vi "Update Status.vi"(9 "Spec Page Interface":T1, 11 "TwoTasksMetaDataObj in":refnum<class "DCAFConfigurablePluginDecideFeatures.lvclass">) -> ()   [LabVIEW 2013, in "DCAFConfigurablePluginDecideFeatures.lvclass"]
uses:
  DCAFConfigurablePluginDecideFeatures.lvclass
  <resource>/dialog/NewProjectWizard/Spec Page Interface.ctl
  <resource>/dialog/NewProjectWizard/MetaDataObj/MetaDataObj.lvclass/MetaDataObj.ctl
  <resource>/dialog/NewProjectWizard/MetaDataObj/Accessors/Read Project Name.vi
  <resource>/dialog/NewProjectWizard/MetaDataObj/Accessors/Read Project Root.vi
  <resource>/dialog/NewProjectWizard/MetaDataObj/Accessors/Read File Prefix.vi
panel:
  in  "Please choose a different name.":string="Please choose a different name."
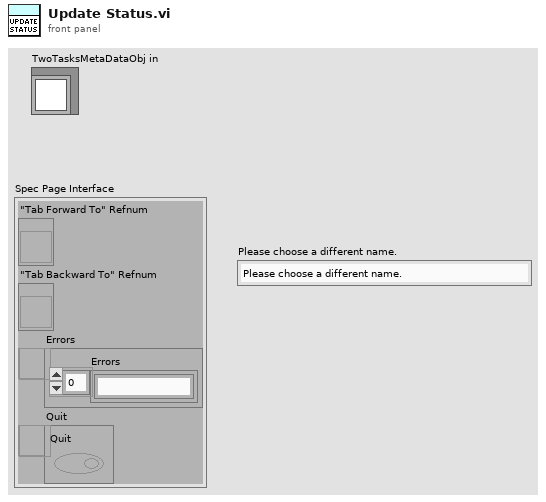
[diagram p1: front panel]
types:
  T1 = typedef "Spec Page Interface.ctl" = cluster{"\"Tab Forward To\" Refnum":refnum<vi>, "\"Tab Backward To\" Refnum":refnum<vi>, "Errors":refnum<user-event>, "Quit":refnum<user-event>}
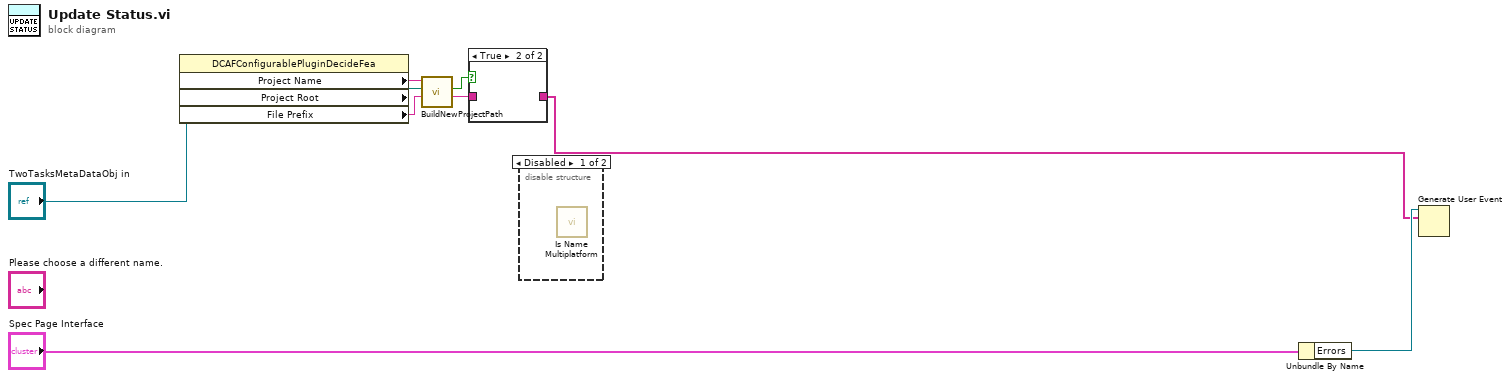
[diagram p0: block diagram]
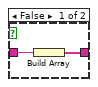
[diagram p3: hidden frame]
diagram:
  n1 = property class="DCAFConfigurablePluginDecideFea"(reference="TwoTasksMetaDataObj in") -> ("Project Name"=w5:string, "Project Root"=w6:path, "File Prefix"=w4:string)  [unwired: 1 in, 2 out]
  n2 = call <resource>:"BuildNewProjectPath.vi"("File Prefix"=w4, "Project Root"=w6, "Project Name"=w5) -> ("Error Message"=w2:string, "Valid?"=w3:bool)  [unwired: 6 in, 1 out]
  n3 = case shown="True" w3 {
    tunnel: w2 -> [w11 _]
    tunnel: [w10 _] -> w1
    frame False {
      n4 = Build Array(w11) -> (w10:string[])
    }
    frame True {
    }
  }
  n5 = disable-structure shown="Disabled" {
    frame Disabled {
      n6 = call <vilib>:"Is Name Multiplatform.vi"() -> ()  [unwired: 7 in, 5 out]
    }
    frame Enabled {
    }
  }
  n7 = Unbundle By Name("Spec Page Interface") -> ("Errors"=w8:refnum<user-event>)
  n8 = Generate User Event(user event=w8, event data cluster=w1) -> ()  [unwired: 2 in, 2 out]
